vi "Write DLL path.vi"(8 "error in (no error)":errorcluster, 10 "DLL path":path, 11 "DelayLine in":refnum<class "DelayLine.lvclass">) -> (0 "error out":errorcluster, 3 "DelayLine out":refnum<class "DelayLine.lvclass">)   [LabVIEW 2015, in "DelayLine.lvclass"]
uses:
  DelayLine.lvclass
  DelayLine.lvclass/DelayLine.ctl
  <vilib>/Utility/error.llb/Error Cluster From Error Code.vi
  <vilib>/ErrorRing/Error Ring.xnode
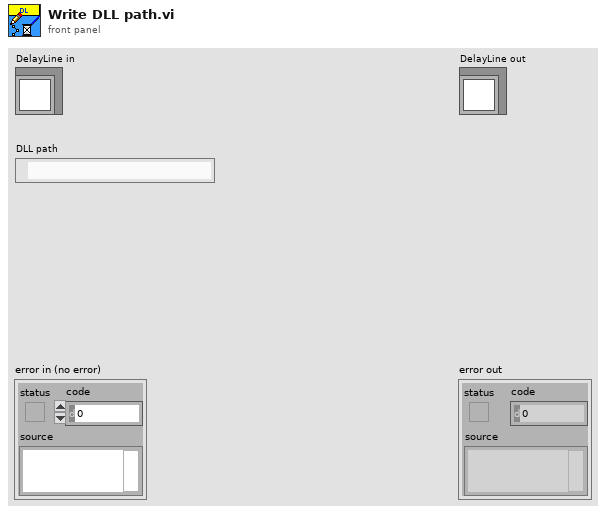
[diagram p1: front panel]
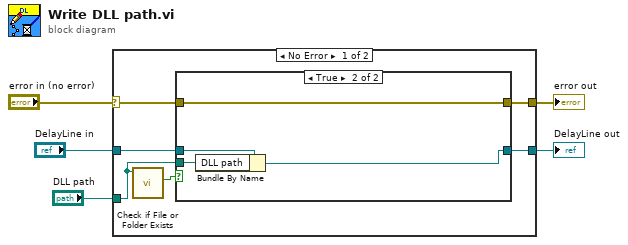
[diagram p0: block diagram]
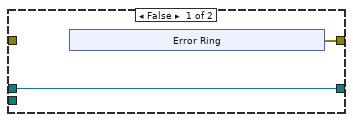
[diagram p2: hidden frame]
diagram:
  n1 = case shown="No Error" "error in (no error)" {
    selector: "error in (no error)" -> [w7 w22]
    tunnel: [w6 w22] -> w4
    tunnel: [w10 w23] -> w2
    tunnel: "DelayLine in" -> [w11 w23]
    tunnel: "DLL path" -> [w8 _]
    frame No Error {
      n2 = call <vilib>:"Check if File or Folder Exists.vi"("path"=w8) -> ("file or folder exists?"=w9:bool)  [unwired: 8 in, 2 out]
      n3 = case shown="True" w9 {
        tunnel: w11 -> [w13 w21]
        tunnel: [w13 w20] -> w10
        tunnel: w8 -> [_ w19]
        tunnel: [w12 w18] -> w6
        tunnel: w7 -> [_ w18]
        frame False {
          n4 = xnode "Error Ring"() -> ("error out"=w12:errorcluster)
        }
        frame True {
          n5 = Bundle By Name(cluster=w21, "DLL path"=w19) -> (w20:refnum<class "DelayLine.lvclass">)
        }
      }
    }
    frame Error {
    }
  }
  "error out" <- w4
  "DelayLine out" <- w2
